vi "Reshape 1D Array__ogtk.vi"(8 "error in (no error)":errorcluster, 9 "Size(s)":u32[](array[numeric]), 10 "1D Array":variant) -> (0 "error out":errorcluster, 2 "Reshaped VArray":variant)   [LabVIEW 2014]
doc: "Reshapes all elements from a 1D array in a variant MultiD array."
uses:
  <userlib>/_OpenG.lib/lvdata/lvdata.llb/Type Descriptor Enumeration__ogtk.ctl
panel:
  # "[OpenG VI Tags] ***Do Not Remove***"
  # "Reshape Array to 1D VArray.vi\n\nReshapes all elements from a 1D array in a variant MultiD array.\n\nPlease visit http://www.OpenG.org to learn about the\nOpen Source LabVIEW software movement.\n\nNOTICE -- YOU MUST LEAVE THIS NOTICE IN PLACE.  PER THE TERMS OF THE LICENSE BELOW, YOU MAY SUBLICENSE THIS SOFTWARE \nIN ANY WAY THAT DOES NOT CONFLICT WITH THIS LICENSE.\n\n### BSD License (http://www.opensource.org/licenses/bsd-license.php) Begin ###\n \nCopyright (c) 2002, Jean-Pierre Drolet <drolet_jp@hotmail.com>\nCopyright (c) 2002-2006, Jim Kring <jim@jimkring.com>\n\nAll rights reserved.\n\nRedistribution and use in source and binary forms, with or without modification, are permitted provided that the following conditions are met:\n\n    * Redistributions of source code must retain the above copyright notice, this list of conditions and the following disclaimer.\n    * Redistributions in binary form must reproduce the above copyright notice, this list of conditions and the following disclaimer in the \n       documentation and/or other materials provided with the distribution.\n    * Neither the name of SciWare, James Kring, Inc., nor the names of its contributors may be used to endorse or promote products derived \n       from this software without specific prior written permission.\n\nTHIS SOFTWARE IS PROVIDED BY THE COPYRIGHT HOLDERS AND CONTRIBUTORS \"AS IS\" AND ANY EXPRESS OR IMPLIED WARRANTIES, \nINCLUDING, BUT NOT LIMITED TO, THE IMPLIED WARRANTIES OF MERCHANTABILITY AND FITNESS FOR A PARTICULAR PURPOSE ARE \nDISCLAIMED. IN NO EVENT SHALL THE COPYRIGHT OWNER OR CONTRIBUTORS BE LIABLE FOR ANY DIRECT, INDIRECT, INCIDENTAL,\n SPECIAL, EXEMPLARY, OR CONSEQUENTIAL DAMAGES (INCLUDING, BUT NOT LIMITED TO, PROCUREMENT OF SUBSTITUTE GOODS OR \nSERVICES; LOSS OF USE, DATA, OR PROFITS; OR BUSINESS INTERRUPTION) HOWEVER CAUSED AND ON ANY THEORY OF LIABILITY, \nWHETHER IN CONTRACT, STRICT LIABILITY, OR TORT (INCLUDING NEGLIGENCE OR OTHERWISE) ARISING IN ANY WAY OUT OF THE USE \nOF THIS SOFTWARE, EVEN IF ADVISED OF THE POSSIBILITY OF SUCH DAMAGE.\n\n### BSD License End ###"
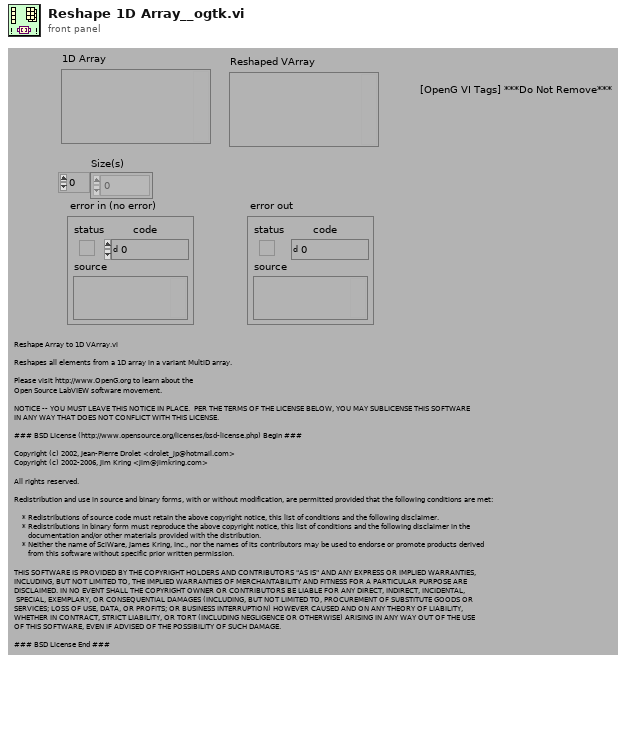
[diagram p1: front panel]
types:
  T1 = typedef "Type Descriptor Enumeration__ogtk.ctl" = enum8{"<Null>", "I8", "I16", "I32", "I64", "U8", "U16", "U32", "U64", "SGL", "DBL", "EXT", "CSG", "CDB", "CXT", "0x0F", "0x10", "0x11", "0x12", "0x13", "0x14", "Enum U8", "Enum U16", "Enum U32", "Enum U64", "SGL PQ", "DBL PQ", "EXT PQ", "CSG PQ", "CDB PQ", "CXT PQ", "0x1F", "0x20", "Boolean", "0x22", "0x23", "0x24", "0x25", "0x26", "0x27", "0x28", "0x29", "0x2A", "0x2B", "0x2C", "0x2D", "0x2E", "0x2F", "String", "0x31", "Path", "Pict", "0x34", "0x35", "0x36", "DAQ", "0x38", "0x39", "0x3A", "0x3B", "0x3C", "0x3D", "0x3E", "0x3F", "Array", "0x41", "0x42", "0x43", "0x44", "0x45", "0x46", "0x47", "0x48", "0x49", "0x4A", "0x4B", "0x4C", "0x4D", "0x4E", "0x4F", "Cluster", "0x51", "0x52", "Variant", "Waveform", "0x55", "0x56", "0x57", "0x58", "0x59", "0x5A", "0x5B", "0x5C", "0x5D", "0x5E", "0x5F", "0x60", "0x61", "0x62", "0x63", "0x64", "0x65", "0x66", "0x67", "0x68", "0x69", "0x6A", "0x6B", "0x6C", "0x6D", "0x6E", "0x6F", "Refnum"}
  T2 = typedef "Type Descriptor Header__ogtk.ctl" = cluster{"length":u16, "private":u8, "type":T1, "# elements":u16}
  T3 = typedef "Type Descriptor__ogtk.ctl" = i16[]
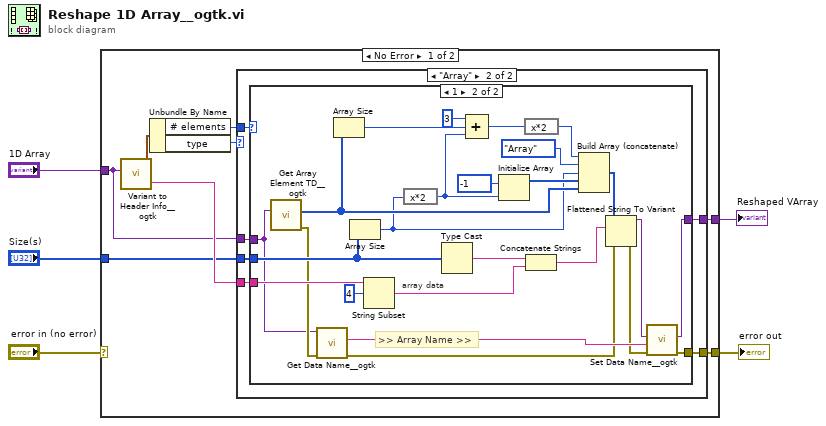
[diagram p0: block diagram]
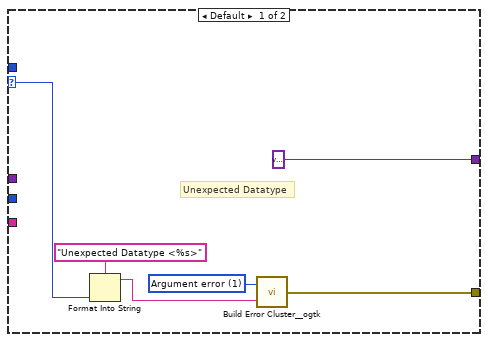
[diagram p2: hidden frame]
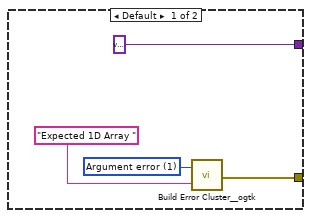
[diagram p3: hidden frame]
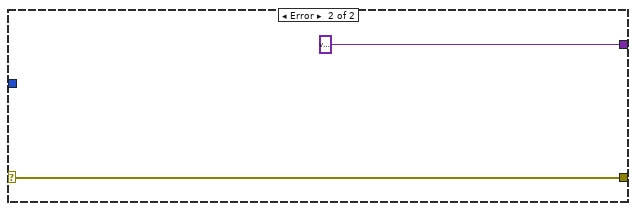
[diagram p4: hidden frame]
diagram:
  n1 = case shown="No Error" "error in (no error)" {
    selector: "error in (no error)" -> [_ w56]
    tunnel: [w13 w56] -> w5
    tunnel: [w8 variant ("Variant")] -> w3
    tunnel: "1D Array" -> [w9 _]
    tunnel: "Size(s)" -> [w7 _]
    frame No Error {
      n2 = call <userlib>:"Variant to Header Info__ogtk.vi"("Variant"=w9) -> ("Type Descriptor Header"=w12:T2, "data string"=w10:string)  [unwired: 3 in, 1 out]
      n3 = Unbundle By Name(w12) -> ("# elements"=w6:u16, "type"=w11:T1)
      n4 = case shown="\"Array\"" w11 {
        selector: w11 -> [w16 _]
        tunnel: [w19 w21] -> w13
        tunnel: w10 -> [_ w25]
        tunnel: w9 -> [_ w22]
        tunnel: [variant ("Variant") w24] -> w8
        tunnel: w7 -> [_ w23]
        tunnel: w6 -> [_ w20]
        frame Default {
          w18 = 1 items=["No error", "Argument error", "Memory is full", "Out of zone", "End of file", "File already open", "Generic file I/O error", "File not found", "File permission error", "Disk is full", "Duplicate path", "Too many files open", "System feature not enabled", "Resource file not found", "Cannot add resource", "Resource not found", "Image not found", "Image memory error", "Pen does not exist", "Config type invalid", "Config token not found", "Config parse error", "Config memory error", "Bad external code format", "Bad external code offset", "External code not present", "Null window", "Destroy window error", "Null menu", "Print aborted", "Bad print record", "Print driver error", "Windows error during printing", "Memory error during printing", "Print dialog error", "Generic print error", "Invalid device refnum", "Device not found", "Device parameter error", "Device unit error", "Cannot open device", "Device call aborted", "Generic error", "Cancelled by user", "Object ID too low", "Object ID too high", "Object not in heap", "Unknown heap", "Unknown object (invalid DefProc)", "Unknown object (DefProc not in table)", "Message out of range", "Invalid (null) method", "Unknown message", "Manager call not supported", "Bad address", "Network operation in progress", "Network operation timed out", "Connection is busy", "Network attribute not supported", "Network error", "Address in use", "System out of memory", "Connection aborted", "Connection refused", "Not connected", "Already connected", "Connection closed", "Initialization error (interapplication manager)", "Bad occurrence", "Wait on unbound occurrence handler", "Occurrence queue overflow", "Datalog type conflict", "Unused", "Unrecognized type (interapplication manager)", "Memory corrupt", "Failed to make temporary DLL", "Old CIN version", "Drag socket not found", "Failed to load drop-object", "Failed to register OLE object", "Failed to release OLE object", "Format specifier type mismatch", "Unknown format specifier", "Too few format specifiers", "Too many format specifiers", "Scan failed", "Newer CIN version", "Error converting to variant", "Runtime menu error", "Password tampered", "Variant attribute not found", "Incompatible variant data type", "Event data is not available", "Event Store is not present", "Occurrence is not found", "Event Queue is not created", "Event info is not available", "Refnum passed is NULL", "Error retrieving Class GUID", "Error retrieving CoClass GUID", "Error retrieving TypeLib GUID.", "Bad built application magic bytes.", "Specific driver is different from the specific driver associated with the Logical Name.", "There is no session opened to the class driver.", "Max Error", "MAX - Error with config objects", "MAX - Error loading configuration", "MAX - Group not supported"]
          # "Unexpected Datatype"
          n5 = Format Into String(format string="Unexpected Datatype <%s>" ("Format String"), w16) -> (resulting string=w14:string)  [unwired: 2 in, 1 out]
          n6 = call <userlib>:"Build Error Cluster__ogtk.vi"("String to Prepend to source (\"\")"=w14, "code"=w18) -> ("error out"=w19:errorcluster)
        }
        frame "Array" {
          n7 = case shown="1" w20 {
            tunnel: w25 -> [_ w53]
            tunnel: [variant ("Variant") w34] -> w24
            tunnel: w23 -> [_ w47]
            tunnel: w22 -> [_ w30]
            tunnel: [w26 w36] -> w21
            frame Default {
              w28 = 1 items=["No error", "Argument error", "Memory is full", "Out of zone", "End of file", "File already open", "Generic file I/O error", "File not found", "File permission error", "Disk is full", "Duplicate path", "Too many files open", "System feature not enabled", "Resource file not found", "Cannot add resource", "Resource not found", "Image not found", "Image memory error", "Pen does not exist", "Config type invalid", "Config token not found", "Config parse error", "Config memory error", "Bad external code format", "Bad external code offset", "External code not present", "Null window", "Destroy window error", "Null menu", "Print aborted", "Bad print record", "Print driver error", "Windows error during printing", "Memory error during printing", "Print dialog error", "Generic print error", "Invalid device refnum", "Device not found", "Device parameter error", "Device unit error", "Cannot open device", "Device call aborted", "Generic error", "Cancelled by user", "Object ID too low", "Object ID too high", "Object not in heap", "Unknown heap", "Unknown object (invalid DefProc)", "Unknown object (DefProc not in table)", "Message out of range", "Invalid (null) method", "Unknown message", "Manager call not supported", "Bad address", "Network operation in progress", "Network operation timed out", "Connection is busy", "Network attribute not supported", "Network error", "Address in use", "System out of memory", "Connection aborted", "Connection refused", "Not connected", "Already connected", "Connection closed", "Initialization error (interapplication manager)", "Bad occurrence", "Wait on unbound occurrence handler", "Occurrence queue overflow", "Datalog type conflict", "Unused", "Unrecognized type (interapplication manager)", "Memory corrupt", "Failed to make temporary DLL", "Old CIN version", "Drag socket not found", "Failed to load drop-object", "Failed to register OLE object", "Failed to release OLE object", "Format specifier type mismatch", "Unknown format specifier", "Too few format specifiers", "Too many format specifiers", "Scan failed", "Newer CIN version", "Error converting to variant", "Runtime menu error", "Password tampered", "Variant attribute not found", "Incompatible variant data type", "Event data is not available", "Event Store is not present", "Occurrence is not found", "Event Queue is not created", "Event info is not available", "Refnum passed is NULL", "Error retrieving Class GUID", "Error retrieving CoClass GUID", "Error retrieving TypeLib GUID.", "Bad built application magic bytes.", "Specific driver is different from the specific driver associated with the Logical Name.", "There is no session opened to the class driver.", "Max Error", "MAX - Error with config objects", "MAX - Error loading configuration", "MAX - Group not supported"]
              n8 = call <userlib>:"Build Error Cluster__ogtk.vi"("String to Prepend to source (\"\")"="Expected 1D Array " ("Format String"), "code"=w28) -> ("error out"=w26:errorcluster)
            }
            frame 1 {
              # ">> Array Name >>"
              # "array data"
              n9 = call <userlib>:"Get Array Element TD__ogtk.vi"("Array"=w30) -> ("error out"=w31:errorcluster, "Type Descriptor"=w44:T3)  [unwired: 9 in]
              n10 = call <userlib>:"Get Data Name__ogtk.vi"("error in (no error)"=w31, "Data"=w30) -> ("error out"=w33:errorcluster, "Data Name"=w37:string)  [unwired: 7 in, 1 out]
              n11 = Array Size(array=w44) -> (size(s)=w43:i32)
              n12 = Array Size(array=w47) -> (size(s)=w39:i32)
              n13 = String Subset(string=w53, offset (0)=4) -> (substring=w51:string)  [unwired: 1 in]
              n14 = expression code="x*2"(w39) -> (w38:i32)
              n15 = Type Cast(x=w47) -> (*(type *) &x=w52:string)  [unwired: 1 in]
              n16 = Compound Arithmetic op=ADD(3 ("Input"), w43, w38) -> (w41:i32)
              n17 = Initialize Array(i16 -1 ("Input Element"), w38) -> (w45:i16[])
              n18 = expression code="x*2"(w41) -> (w40:i32)
              n19 = Concatenate Strings(w52, w51) -> (w49:string)
              n20 = Build Array (concatenate)(w40, Type_Descriptor_Enumeration__ogtk."Array" ("Type Descriptor Enumeration"), w39, w45, w44) -> (w50:i32[])
              n21 = Flattened String To Variant(4:w33, 6:w49, 7:w50) -> (0:w32:errorcluster, 3:w35:variant)
              n22 = call <userlib>:"Set Data Name__ogtk.vi"("error in (no error)"=w32, "Data Name"=w37, "Data"=w35) -> ("error out"=w36:errorcluster, "Renamed Data"=w34:variant)  [unwired: 7 in]
            }
          }
        }
      }
    }
    frame Error {
    }
  }
  "error out" <- w5
  "Reshaped VArray" <- w3
